vi "Timer.vi"(7 "Method":T1(ring)=enum."Get Elapsed Time", 8 "error in (no error)":errorcluster, 10 "Timeout":dbl, 11 "BehaviorData in":refnum<class "TrialBasedExperiment.lvclass">) -> (0 "error out":errorcluster, 1 "Timeout":bool, 2 "Time":dbl, 3 "BehaviorData out":refnum<class "TrialBasedExperiment.lvclass">)   [LabVIEW 2011, in "TrialBasedExperiment.lvclass"]
uses:
  TrialBasedExperiment.lvclass
  Acquisition/BehaviorData/BehaviorData.lvclass
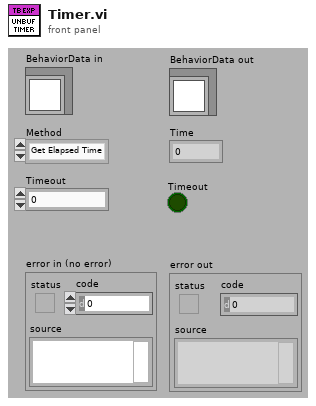
[diagram p1: front panel]
types:
  T1 = enum16{"Get Time", "Get Elapsed Time", "Reset Elapsed Time"}
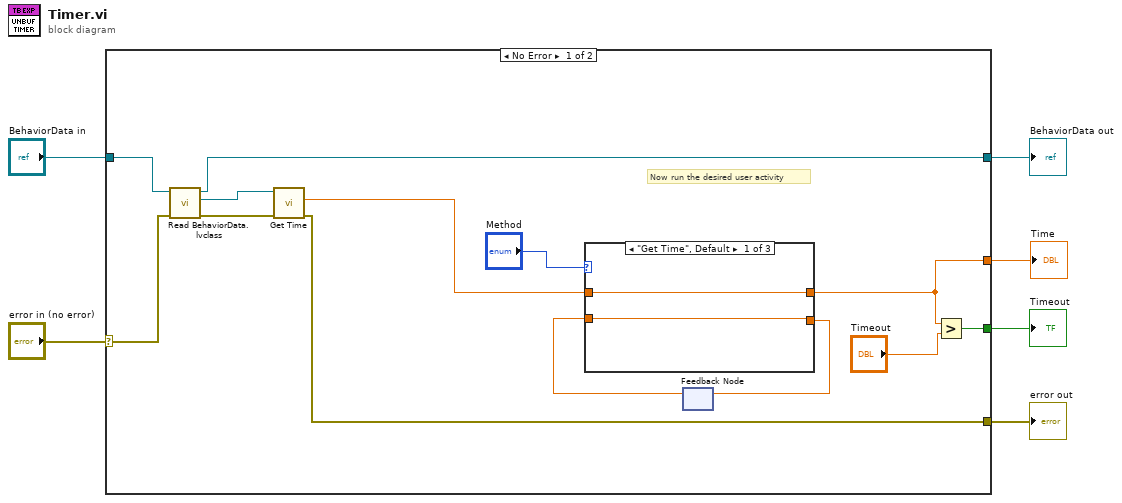
[diagram p0: block diagram]
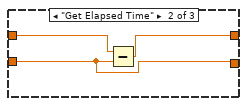
[diagram p2: hidden frame]
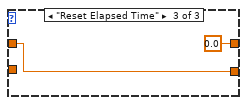
[diagram p3: hidden frame]
diagram:
  n1 = case shown="No Error" "error in (no error)" {
    selector: "error in (no error)" -> [w8 w28]
    tunnel: [w7 w28] -> w5
    tunnel: [w10 w27] -> w3
    tunnel: "BehaviorData in" -> [w11 w27]
    tunnel: [w16 _] -> w2
    tunnel: [w14 _] -> w1
    frame No Error {
      # "Now run the desired user activity"
      n2 = call-dynamic "Read BehaviorData.lvclass.vi"("error in (no error)"=w8, "TrialBasedExperiment in"=w11) -> ("error out"=w12:errorcluster, "BehaviorData.lvclass"=w13:refnum<class "BehaviorData.lvclass">, "TrialBasedExperiment out"=w10:refnum<class "TrialBasedExperiment.lvclass">)  [unwired: 7 in]
      n3 = call-dynamic "Get Time.vi"("error in (no error)"=w12, "BehaviorData in"=w13) -> ("error out"=w7:errorcluster, "Counter Time"=w9:dbl)  [unwired: 7 in, 1 out]
      n4 = feedback #1() -> (w18:dbl)  [unwired: 1 in]
      n5 = case shown="\"Get Time\", Default" "Method" {
        tunnel: w9 -> [w21 w24 w26]
        tunnel: [w21 w23 0.0] -> w16
        tunnel: w18 -> [w20 w22 _]
        tunnel: [w20 w22 w26] -> w17
        frame "Get Time", Default {
        }
        frame "Get Elapsed Time" {
          n6 = Subtract(x=w24, y=w22) -> (x-y=w23:dbl)
        }
        frame "Reset Elapsed Time" {
        }
      }
      n7 = feedback-in #1(w17) -> ()
      n8 = Greater?(x=w16, y="Timeout") -> (0:w14:bool)
    }
    frame Error {
    }
  }
  "error out" <- w5
  "BehaviorData out" <- w3
  "Time" <- w2
  "Timeout" <- w1
